vi "Get Timestamp.vi"() -> (3 "Timestamp":string)   [LabVIEW 2020]
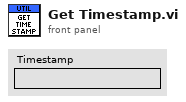
[diagram p1: front panel]
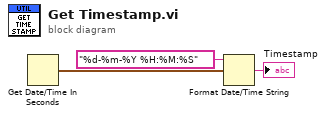
[diagram p0: block diagram]
diagram:
  n1 = Get Date/Time In Seconds() -> (seconds since 1Jan1904=w3:timestamp)
  n2 = Format Date/Time String(time format string (%c)="%d-%m-%Y %H:%M:%S", seconds (now)=w3) -> (date/time string=→"Timestamp":string)  [unwired: 1 in]
